vi "Stop.vi"(8 "Error In":errorcluster, 11 "object in":refnum<class "Rigol DS1054.lvclass">) -> (0 "Error Out":errorcluster, 3 "object out":refnum<class "Rigol DS1054.lvclass">)   [LabVIEW 2023, in "RIGOL DS1054Z.lvlib" / "Rigol DS1054.lvclass"]
uses:
  Rigol DS1054.lvclass
  <instrlib>/RIGOL-DS1054Z-LabVIEW/RIGOL DS1054Z Driver.lvlib
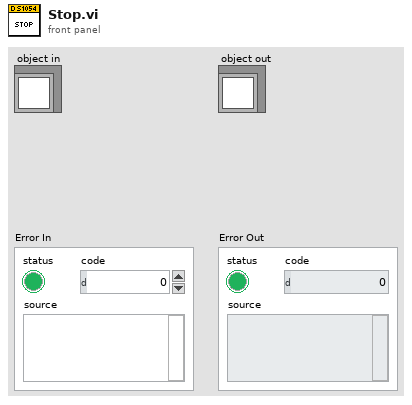
[diagram p1: front panel]
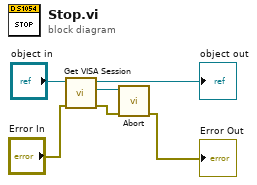
[diagram p0: block diagram]
diagram:
  n1 = call-dynamic "Get VISA Session.vi"("error in"="Error In", "Scope VISA in"="object in") -> ("error out"=w4:errorcluster, "VISA session"=w3:refnum<visa-resource-name>, "Scope VISA out"=→"object out":refnum<class "Rigol DS1054.lvclass">)  [unwired: 7 in]
  n2 = call <instrlib>:"Abort.vi"("error in (no error)"=w4, "VISA resource name"=w3) -> ("error out"=→"Error Out":errorcluster)  [unwired: 8 in, 1 out]
